vi "Get Module Info.vi"(8 "error in":errorcluster, 11 "Module Detection in":refnum<class "Module Detection.lvclass">) -> (0 "error out":errorcluster, 2 "Module Info":T1[](array[typedef]) {"Product ID" format="%.0x"}, 3 "Module Detection out":refnum<class "Module Detection.lvclass">)   [LabVIEW 2015]
uses:
  SysCfg Device/SysCfg Device.lvclass
  Module Detection.lvclass
  Distributed Devices/Controls/DeviceInformation.ctl
  Distributed Devices/Device.lvclass
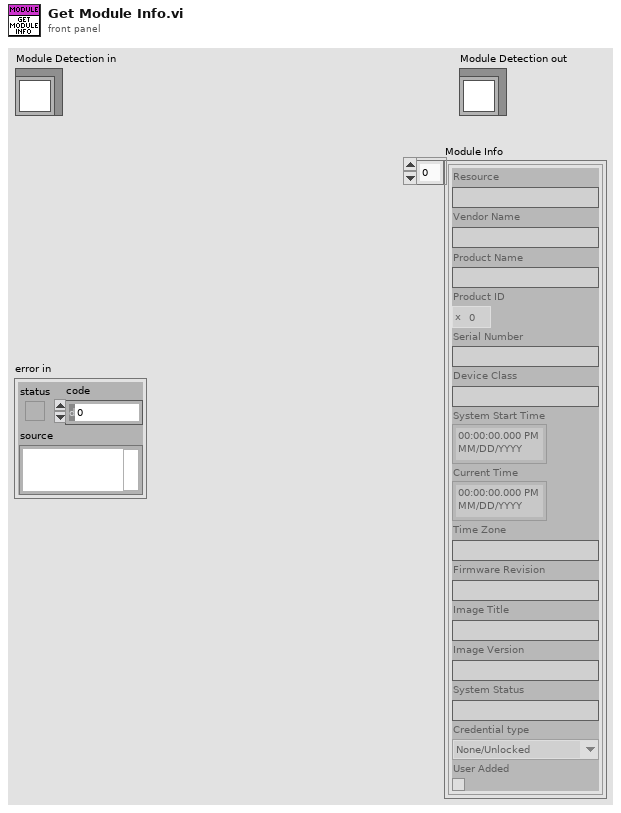
[diagram p1: front panel]
types:
  T1 = typedef "SMI.lvlib/Device.lvclass/DeviceInformation.ctl" = cluster{"Resource":string, "Vendor Name":string, "Product Name":string, "Product ID":u32, "Serial Number":string, "Device Class":string, "System Start Time":timestamp, "Current Time":timestamp, "Time Zone":string, "Firmware Revision":string, "Image Title":string, "Image Version":string, "System Status":string, "Credential type":enum16{"None/Unlocked", "FTP Password", "NIAuth Credentials"}, "User Added":bool}
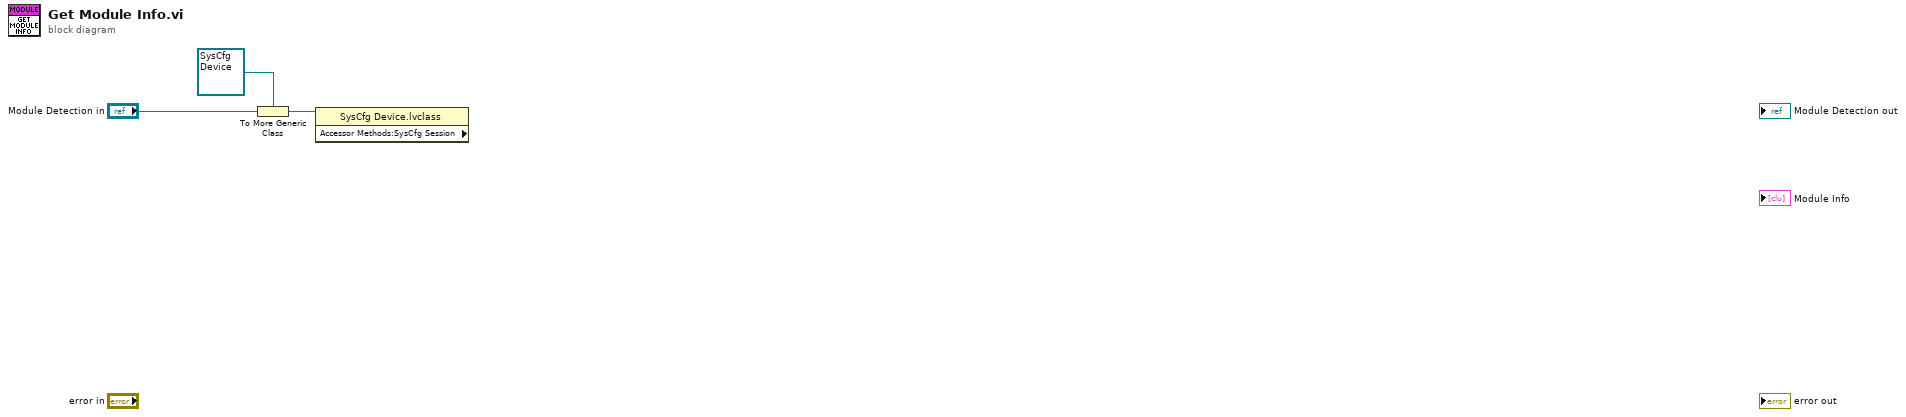
[diagram p0: block diagram]
diagram:
  n1 = To More Generic Class(target class=refnum<class "SysCfg Device.lvclass"> refnum ("SMI.lvlib:SysCfg Device.lvclass"), reference="Module Detection in") -> (generic class reference=w2:refnum<class "SysCfg Device.lvclass">)
  n2 = property class="SysCfg Device.lvclass" props=["Accessor Methods:SysCfg Session"](reference=w2) -> ()  [unwired: 1 in, 3 out]
